vi "Change VI Icon.vi"(8 "Error In":errorcluster, 9 "Icon Colors":T2={"Text Color"=0, "Background Color"=16448250, "Border Color"=16746744}, 10 "Icon Text":T1={"Line 1 text"="Bus", "Line 2 text"="Dev", "Line 3 text"="Ch", "Line 4 text"=""}, 11 "Reference to VI In":refnum<vi>) -> (0 "Error Out":errorcluster, 3 "Reference to VI Out":refnum<vi>)   [LabVIEW 2014]
doc: "Creates a VI Icon with up to 4 lines of text and applies it to the VI that has its reference is inputted."
uses:
  Icon Editor/Icon Editor.llb/Icon Colors.ctl
  <vilib>/LabVIEW Icon API/API_Text.ctl
  <vilib>/LabVIEW Icon API/LabVIEW Icon API.lvlib
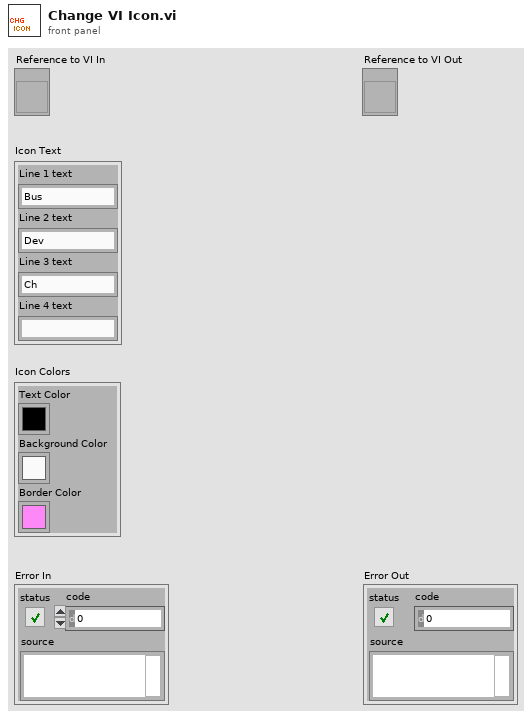
[diagram p1: front panel]
types:
  T1 = typedef "LabVIEW Icon API.lvlib/API_Text.ctl" = cluster{"Line 1 text":string, "Line 2 text":string, "Line 3 text":string, "Line 4 text":string}
  T2 = typedef "Icon Colors.ctl" = cluster{"Text Color":u32, "Background Color":u32, "Border Color":u32}
  T3 = cluster{"left":i16, "top":i16, "right":i16, "bottom":i16}
  T4 = typedef "imagedata.ctl" = cluster{"image type":i32, "image depth":i32, "image":u8[], "mask":u8[], "colors":u32[], "Rectangle":cluster{"left":i16, "top":i16, "right":i16, "bottom":i16}}
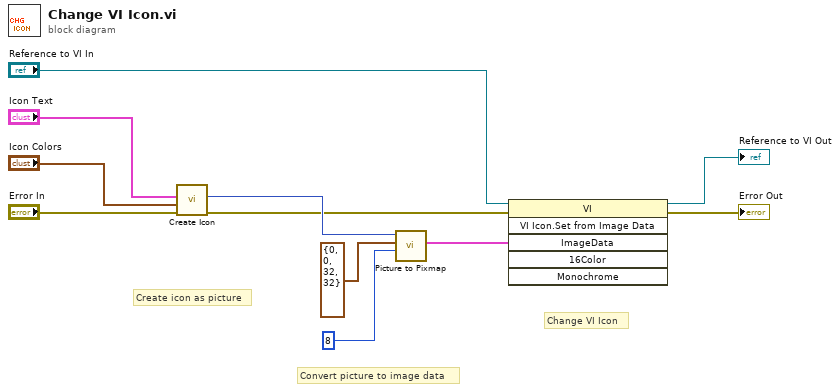
[diagram p0: block diagram]
diagram:
  # "Create icon as picture"
  # "Change VI Icon"
  # "Convert picture to image data"
  n1 = call "Create Icon.vi"("error in"="Error In", "Icon Colors"="Icon Colors", "Icon Text"="Icon Text") -> ("error out"=w8:errorcluster, "Picture"=w10:picture)  [unwired: 7 in]
  n2 = call <vilib>:"Picture to Pixmap.vi"("depth"=8, "rect"=T3 {"left"=0, "top"=0, "right"=32, "bottom"=32}, "picture"=w10) -> ("image data"=w3:T4)  [unwired: 7 in, 1 out]
  n3 = invoke class="VI" method="VI Icon.Set from Image Data"(reference="Reference to VI In", error in=w8, "ImageData"=w3) -> (reference out=→"Reference to VI Out":refnum<vi>, error out=→"Error Out":errorcluster)  [unwired: 3 in, 4 out]
